vi "Write ROI XY.vi"(8 "error in (no error)":errorcluster, 10 "ROI XY":T1, 11 "TG Base Graph in":refnum<class "Base Graph.lvclass">) -> (0 "error out":errorcluster, 3 "TG Base Graph out":refnum<class "Base Graph.lvclass">)   [LabVIEW 2023, in "Base Graph.lvclass"]
uses:
  Base Graph.lvclass
  Base Graph.lvclass/Base Graph.ctl
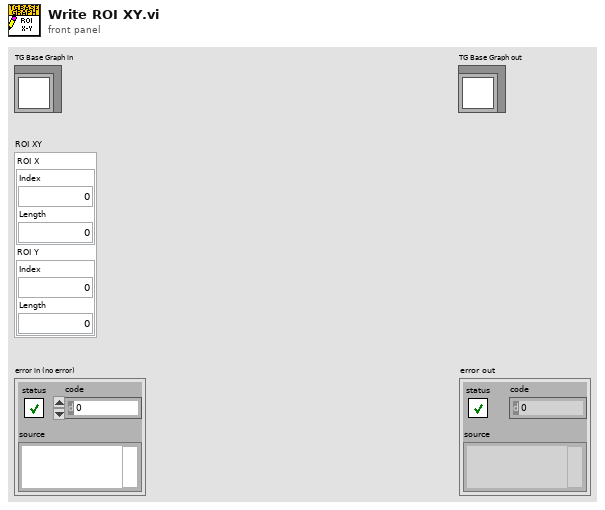
[diagram p1: front panel]
types:
  T1 = cluster{"ROI X":cluster{"Index":u32, "Length":u32}, "ROI Y":cluster{"Index":u32, "Length":u32}}
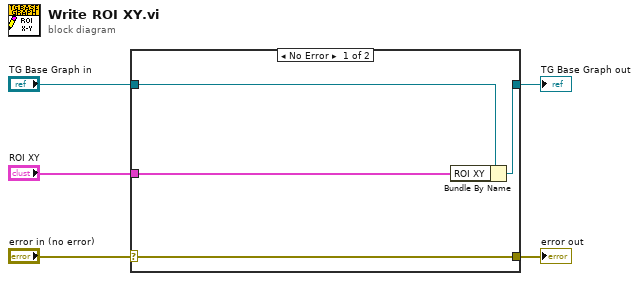
[diagram p0: block diagram]
diagram:
  n1 = case shown="No Error" "error in (no error)" {
    selector: "error in (no error)" -> [w9 w10]
    tunnel: [w9 w10] -> w4
    tunnel: [w7 w11] -> w2
    tunnel: "TG Base Graph in" -> [w8 w11]
    tunnel: "ROI XY" -> [w6 _]
    frame No Error {
      n2 = Bundle By Name(cluster=w8, "ROI XY"=w6) -> (w7:refnum<class "Base Graph.lvclass">)
    }
    frame Error {
    }
  }
  "error out" <- w4
  "TG Base Graph out" <- w2
